vi "SetClassQueueMessage.vi"(8 "ErrorIn(No Error)":errorcluster caption="entrée d'erreur (pas d'erreur)", 10 "Menu déroulant":T1 items=["UpdateClassData", "UpdateMainClass"], 11 "PhotoLum.lvclass":refnum<class "PhotoLum.lvclass">) -> (0 "sortie d'erreur":errorcluster, 3 "PhotoLum.lvclass Out":refnum<class "PhotoLum.lvclass">)   [LabVIEW 2019, in "PhotoLum.lvclass"]
uses:
  PhotoLum.lvclass
  BaseDevice/ClassQueueMess.ctl
  BaseDevice/BaseDevice.lvclass
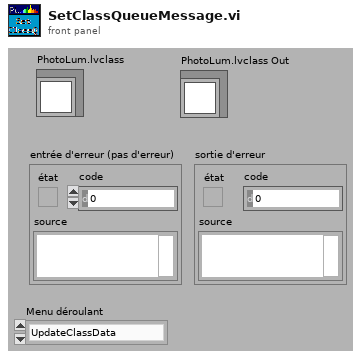
[diagram p1: front panel]
types:
  T1 = typedef "ClassQueueMess.ctl" = u16
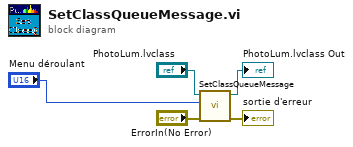
[diagram p0: block diagram]
diagram:
  n1 = call-parent "SetClassQueueMessage.vi"("ErrorIn(No Error)"="ErrorIn(No Error)", "Menu déroulant"="Menu déroulant", "BaseDevice.lvclass"="PhotoLum.lvclass") -> ("sortie d'erreur"=→"sortie d'erreur":errorcluster, "BaseDevice.lvclass Out"=→"PhotoLum.lvclass Out":refnum<class "PhotoLum.lvclass">)  [unwired: 7 in]
